vi "frequency_sweep_1.vi"() -> ()   [LabVIEW 2016]
uses:
  <instrlib>/niVNA/niVNA.llb/niVNA Fetch Sweep Measurement (DBL).vi
panel:
  in  "IF Bandwidth":dbl(ring)=1000.0 items=["10 Hz"=10.0, "30 Hz"=30.0, "100 Hz"=100.0, "300 Hz"=300.0, "1 KHz"=1000.0, "3 KHz"=3000.0, "10 KHz"=10000.0, "30 KHz"=30000.0]
  in  "Save Button":bool
  out "Status":string="Measurement Running..."
  out "Cursor":cluster{"x":dbl, "y":dbl} {"x" format="%.5f"; "y" format="%.5f"}
  out "Resource Name Out":refnum<k15>
  out "Error Out":errorcluster
  in  "Error In (no error)":errorcluster
  in  "Format":i32(ring) items=["Log Magnitude (dB)"=0, "Lin Magnitude"=1, "Phase (deg)"=2, "VSWR"=3, "Group Delay"=6]
  out "SpectrumGraph":cluster{"Numeric":dbl, "real":dbl}[](graph)
  in  "Value":i32(ring)=1 items=["Im", "Re", "Abs"]
  in  "S-parameter":i32(ring)=1 caption="Measurement" items=["S11", "S21"]
  in  "Exit Button":bool
  in  "Start Button":bool
  in  "Stop Button":bool
  in  "Output Power":dbl=1.0
  in  "Number of Points":i32=1024 min=1 max=3201
  in  "Stop Frequency":dbl=6000000000.0 min=10000000.0 max=6000000000.0 format="%#_6e"
  in  "Start Frequency":dbl=1000000000.0 min=10000000.0 max=6000000000.0 format="%#_6e"
  in  "Resource Name In":refnum<k15>="VNA_5630"
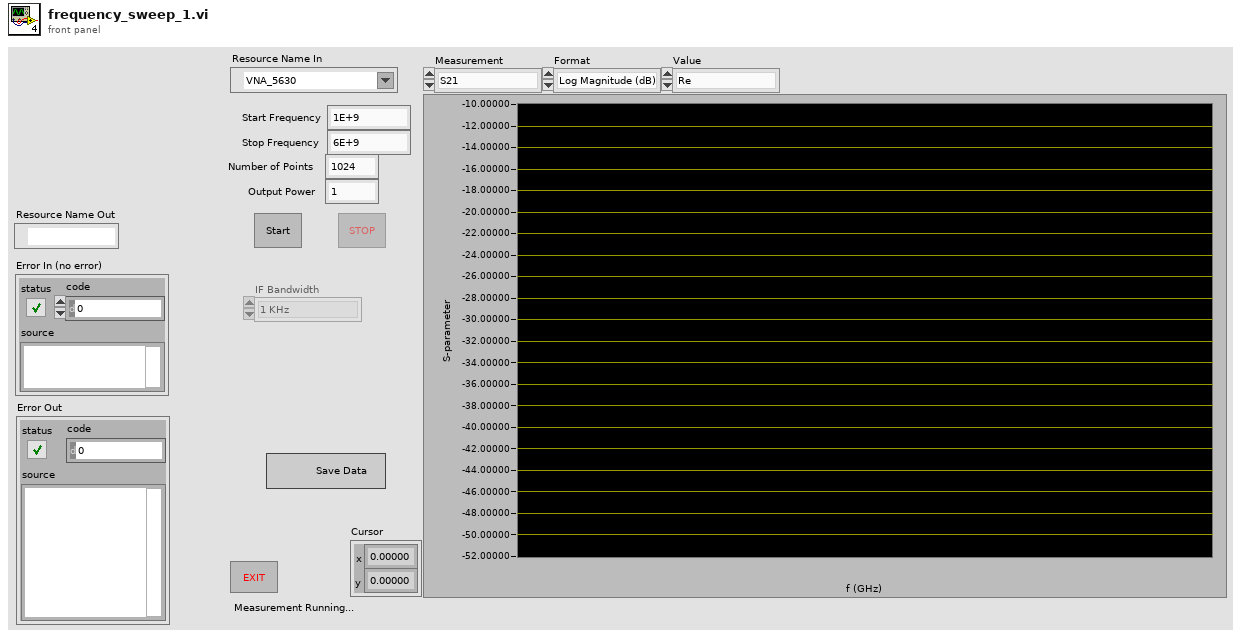
[diagram p1: front panel]
types:
  T1 = typedef "LVPoint32TypeDef.ctl" = cluster{"Horizontal":i32, "Vertical":i32}
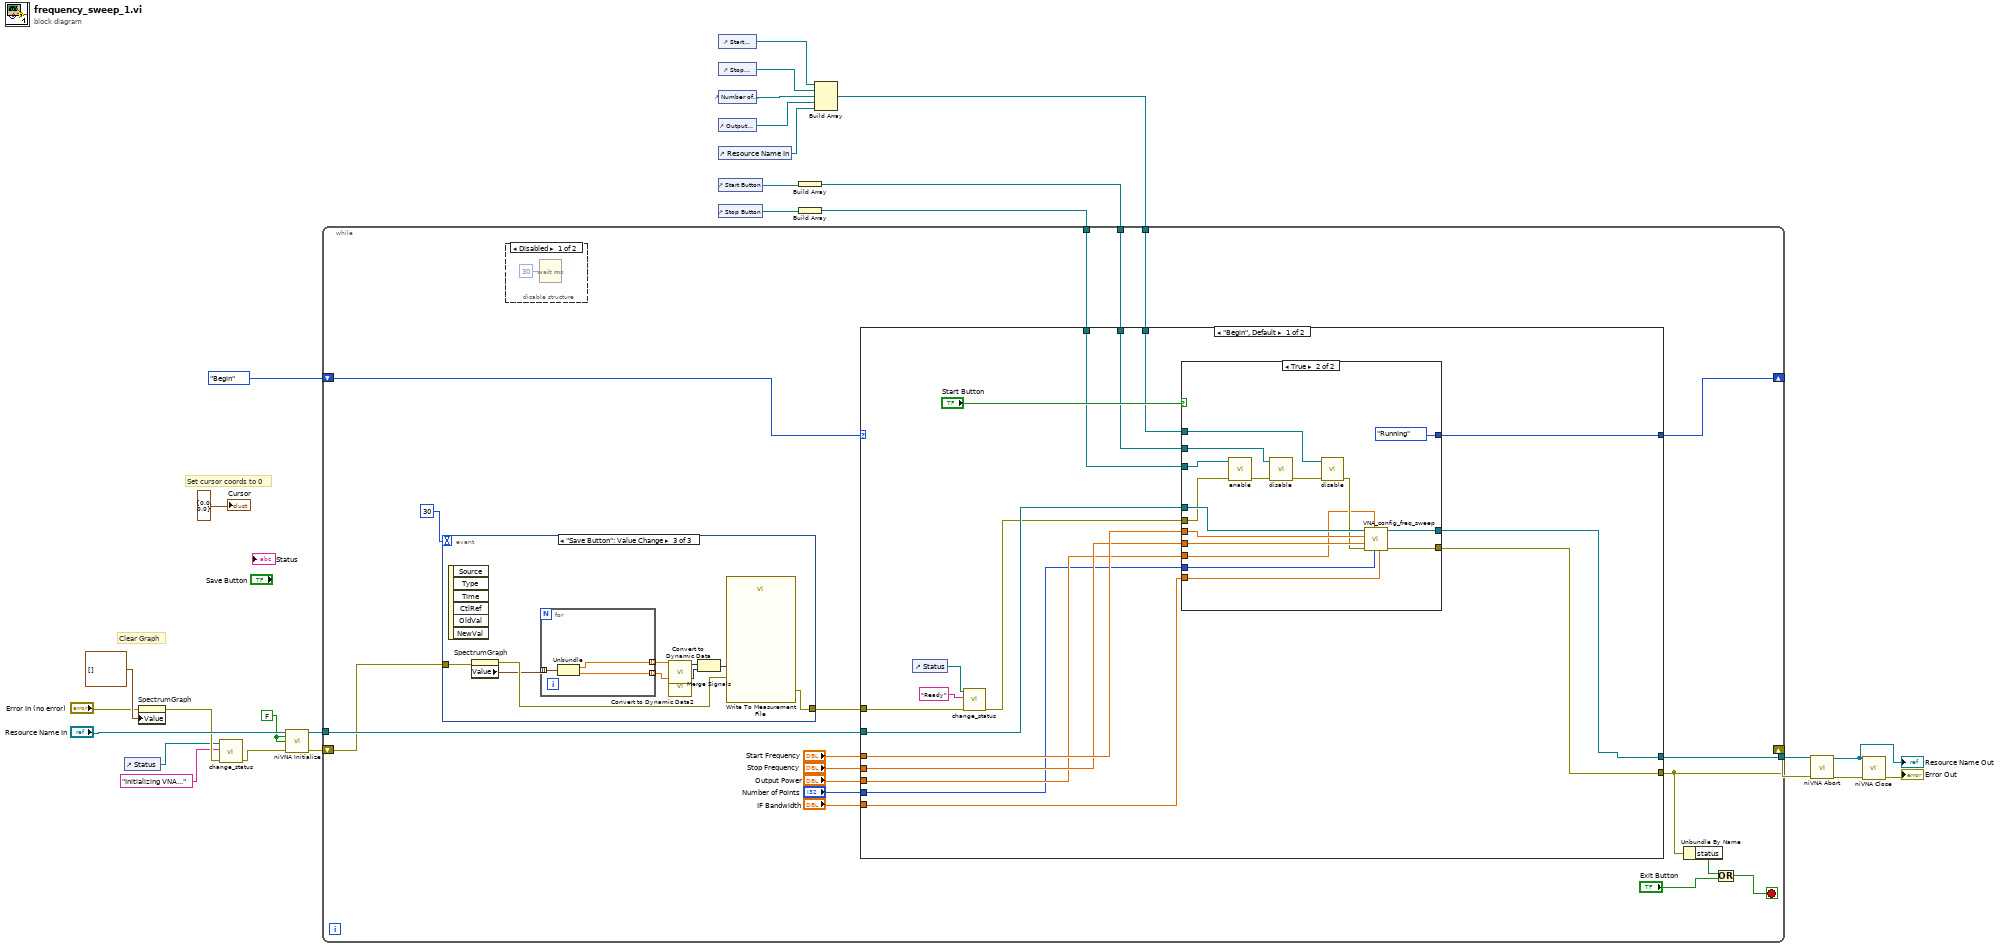
[diagram p0: block diagram]
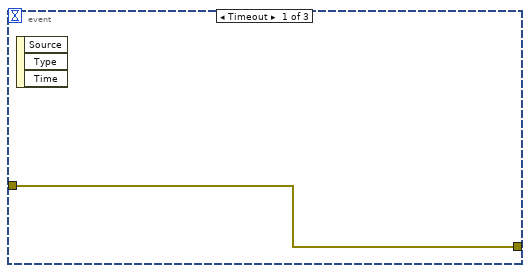
[diagram p3: hidden frame]
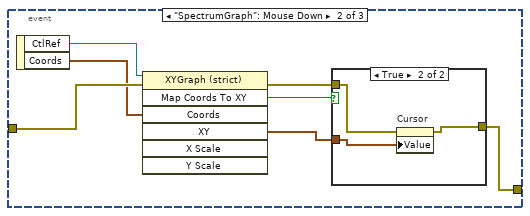
[diagram p4: hidden frame]
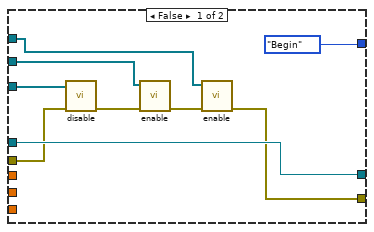
[diagram p6: hidden frame]
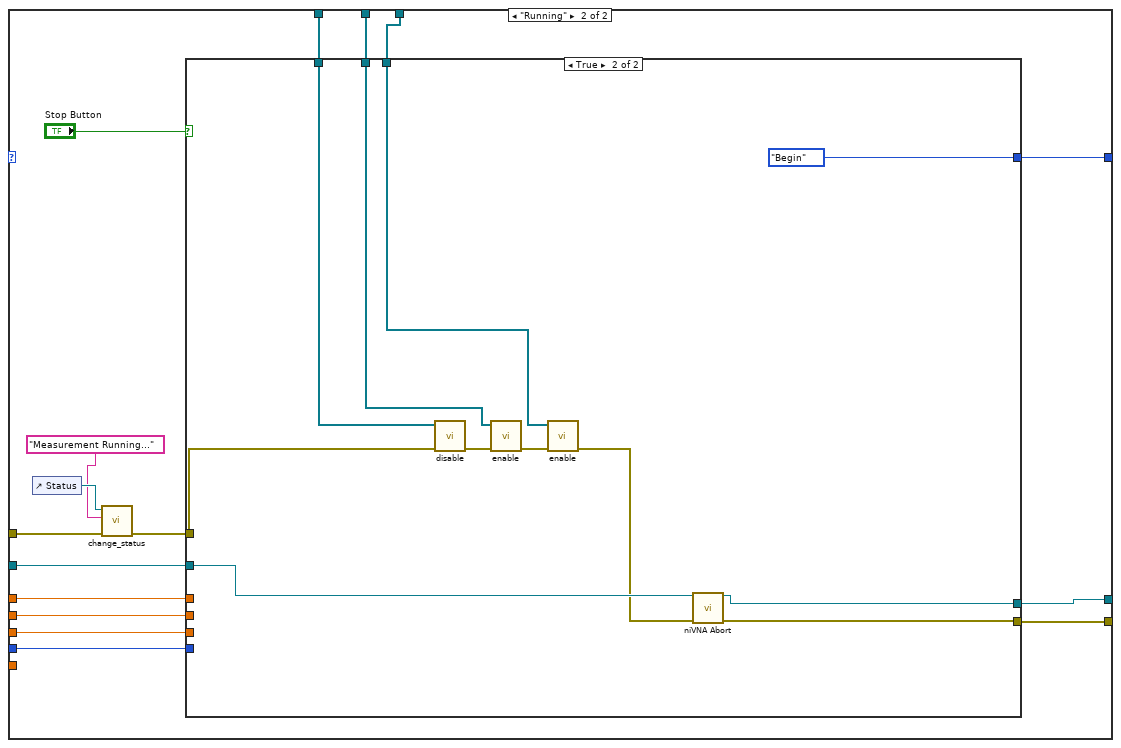
[diagram p7: hidden frame]
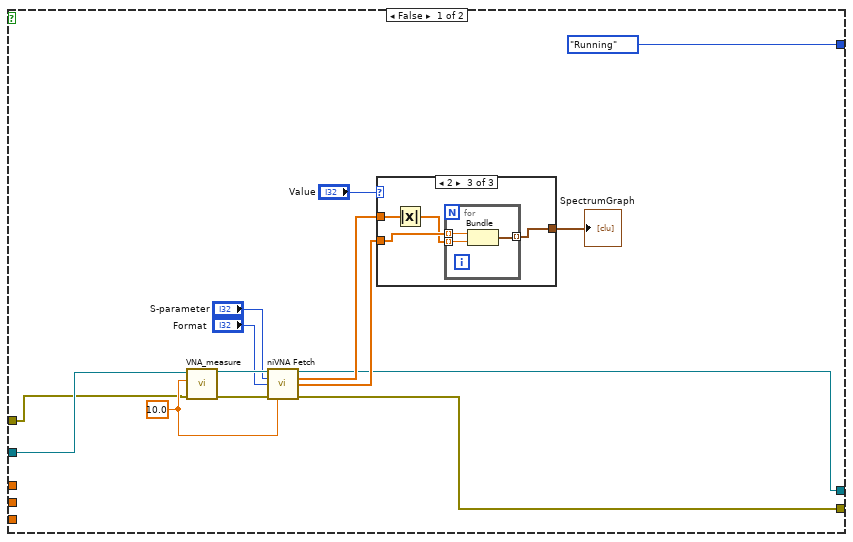
[diagram p8: hidden frame]
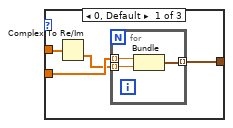
[diagram p9: hidden frame]
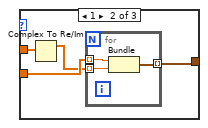
[diagram p10: hidden frame]
diagram:
  w7 = FALSE ("id query")
  # "Set cursor coords to 0"
  # "Clear Graph"
  n1 = control-ref of="Status"() -> (w1:refnum<vi>)
  n2 = property on="SpectrumGraph" class="XYGraph (strict)"(error in="Error In (no error)", "Value"=cluster{"Numeric":dbl, "real":dbl}[] [] ("SpectrumGraph")) -> (error out=w4:errorcluster)  [unwired: 1 in, 1 out]
  n3 = call "change_status.vi"("error in (no error)"=w4, "String"="Initializing VNA...", "String in"=w1) -> ("error out"=w3:errorcluster)  [unwired: 8 in]
  n4 = call <instrlib>:"niVNA Initialize.vi"("resource name"="Resource Name In", "id query"=w7, "reset"=w7, "error in"=w3) -> ("instrument handle"=w8:refnum<k15>, "error out"=w5:errorcluster)  [unwired: 10 in]
  n5 = control-ref of="Start Frequency"() -> (w27:refnum<vi>)
  n6 = control-ref of="Stop Frequency"() -> (w26:refnum<vi>)
  n7 = control-ref of="Number of Points"() -> (w25:refnum<vi>)
  n8 = control-ref of="Output Power"() -> (w24:refnum<vi>)
  n9 = control-ref of="Resource Name In"() -> (w23:refnum<vi>)
  n10 = control-ref of="Start Button"() -> (w19:refnum<vi>)
  n11 = control-ref of="Stop Button"() -> (w21:refnum<vi>)
  n12 = Build Array(w19) -> (w18:refnum<vi>[])
  n13 = Build Array(w21) -> (w20:refnum<vi>[])
  n14 = Build Array(w27, w26, w25, w24, w23) -> (w17:refnum<vi>[])
  n15 = while {
    shift-right: [w41] -> _
    shift-left: enum16{"Begin", "Running"}."Begin" -> [w46]
    tunnel: w20 -> [w37]
    tunnel: w18 -> [w35]
    tunnel: w17 -> [w34]
    tunnel: w8 -> [w33]
    tunnel: [w30] -> w6
    shift-right: [w36] -> w11
    shift-left: w5 -> [w29]
    stop <- w38 stop-if-true
    n16 = event shown="[2] \"Save Button\": Value Change" {
      selector: _ -> [_ _ _]
      dyn-events: _ -> [_ _ _]
      timeout: u32 30 ("milliseconds to wait") -> [_ _ _]
      tunnel: w29 -> [w48 w52 w67]
      tunnel: [w48 w51 w68] -> w32
      event Timeout {
        n17 = event-data() -> ()  [unwired: 1 in, 3 out]
      }
      event "SpectrumGraph": Mouse Down {
        n18 = event-data() -> ("CtlRef"=w49:refnum<vi>, "Coords"=w50:T1)  [unwired: 1 in]
        n19 = invoke on="Invoke Node" class="XYGraph (strict)" method="Map Coords To XY"(reference=w49, error in=w52, "Coords"=w50) -> (error out=w55:errorcluster, "Map Coords To XY"=w53:bool, "XY"=w54:cluster{"X":dbl, "Y":dbl})  [unwired: 4 in, 4 out]
        n20 = case shown="True" w53 {
          tunnel: w54 -> [_ w57]
          tunnel: w55 -> [w56 w59]
          tunnel: [w56 w58] -> w51
          frame False {
          }
          frame True {
            n21 = property on="Cursor" class="Clust (strict)"(error in=w59, "Value"=w57) -> (error out=w58:errorcluster)  [unwired: 1 in, 1 out]
          }
        }
      }
      event "Save Button": Value Change {
        n22 = event-data() -> ()  [unwired: 1 in, 6 out]
        n23 = property on="SpectrumGraph" class="XYGraph (strict)"(error in=w67) -> (error out=w66:errorcluster, "Value"=w65:cluster{"Numeric":dbl, "real":dbl}[])  [unwired: 1 in, 1 out]
        n24 = for {
          tunnel: w65 -> [w71] mode=indexing
          tunnel: [w70] -> w64 mode=indexing
          tunnel: [w69] -> w61 mode=indexing
          n25 = Unbundle(w71) -> ("Numeric"=w70:dbl, "real"=w69:dbl)
        }
        n26 = call "Convert to Dynamic Data"("Array"=w64) -> ("Dynamic Data Type"=w63:dynamicdata)  [unwired: 3 in]
        n27 = call "Convert to Dynamic Data2"("Array"=w61) -> ("Dynamic Data Type"=w60:dynamicdata)  [unwired: 3 in]
        n28 = Merge Signals(w63, w60) -> (w62:dynamicdata)
        n29 = call "Write To Measurement File"("Signals"=w62, "error in (no error)"=w66) -> ("error out"=w68:errorcluster)  [unwired: 15 in, 2 out]
      }
    }
    n30 = disable-structure shown="Disabled" {
      frame Disabled {
        n31 = Wait (ms)(milliseconds to wait=u32 30) -> ()  [unwired: 1 out]
      }
      frame Enabled {
      }
    }
    n32 = case shown="\"Begin\", Default" w46 {
      tunnel: w33 -> [w86 w127]
      tunnel: "Start Frequency" -> [w85 w126]
      tunnel: "Stop Frequency" -> [w84 w125]
      tunnel: "Output Power" -> [w83 w124]
      tunnel: "Number of Points" -> [w82 w123]
      tunnel: [w87 w128] -> w41
      tunnel: [w81 w121] -> w30
      tunnel: [w80 w122] -> w36
      tunnel: w37 -> [w79 w120]
      tunnel: w32 -> [w74 w115]
      tunnel: w35 -> [w78 w119]
      tunnel: w34 -> [w77 w118]
      tunnel: "IF Bandwidth" -> [w72 _]
      frame "Begin", Default {
        n33 = control-ref of="Status"() -> (w75:refnum<vi>)
        n34 = call "change_status.vi"("error in (no error)"=w74, "String"="Ready", "String in"=w75) -> ("error out"=w73:errorcluster)  [unwired: 8 in]
        n35 = case shown="True" "Start Button" {
          tunnel: [enum16{"Begin", "Running"}."Begin" enum16{"Begin", "Running"}."Running"] -> w87
          tunnel: w86 -> [w96 w112]
          tunnel: w85 -> [_ w111]
          tunnel: w84 -> [_ w110]
          tunnel: w83 -> [_ w99]
          tunnel: w82 -> [_ w109]
          tunnel: [w96 w108] -> w81
          tunnel: [w92 w107] -> w80
          tunnel: w79 -> [w95 w102]
          tunnel: w73 -> [w91 w101]
          tunnel: w78 -> [w90 w104]
          tunnel: w77 -> [w89 w103]
          tunnel: w72 -> [_ w98]
          frame False {
            n36 = call "disable.vi"("error in (no error)"=w91, "Array"=w95) -> ("error out"=w94:errorcluster)  [unwired: 9 in]
            n37 = call "enable.vi"("error in (no error)"=w94, "Array"=w90) -> ("error out"=w93:errorcluster)  [unwired: 9 in]
            n38 = call "enable.vi"("error in (no error)"=w93, "Array"=w89) -> ("error out"=w92:errorcluster)  [unwired: 9 in]
          }
          frame True {
            n39 = call "enable.vi"("error in (no error)"=w101, "Array"=w102) -> ("error out"=w100:errorcluster)  [unwired: 9 in]
            n40 = call "disable.vi"("error in (no error)"=w100, "Array"=w104) -> ("error out"=w106:errorcluster)  [unwired: 9 in]
            n41 = call "disable.vi"("error in (no error)"=w106, "Array"=w103) -> ("error out"=w105:errorcluster)  [unwired: 9 in]
            n42 = call "VNA_config_freq_sweep.vi"("IF Bandwidth"=w98, "Number of Points"=w109, "Output Power"=w99, "error in (no error)"=w105, "Stop Frequency"=w110, "Start Frequency"=w111, "Resource Name In"=w112) -> ("error out"=w107:errorcluster, "Resource Name Out"=w108:refnum<k15>)  [unwired: 3 in]
          }
        }
      }
      frame "Running" {
        n43 = control-ref of="Status"() -> (w117:refnum<vi>)
        n44 = call "change_status.vi"("error in (no error)"=w115, "String"="Measurement Running...", "String in"=w117) -> ("error out"=w114:errorcluster)  [unwired: 8 in]
        n45 = case shown="True" "Stop Button" {
          tunnel: [enum16{"Begin", "Running"}."Running" enum16{"Begin", "Running"}."Begin"] -> w128
          tunnel: w127 -> [w134 w174]
          tunnel: w126 -> [_ _]
          tunnel: w125 -> [_ _]
          tunnel: w124 -> [_ _]
          tunnel: w123 -> [_ _]
          tunnel: [w131 w165] -> w122
          tunnel: [w133 w173] -> w121
          tunnel: w114 -> [w130 w167]
          tunnel: w120 -> [_ w170]
          tunnel: w119 -> [_ w169]
          tunnel: w118 -> [_ w168]
          frame False {
            w139 = 10.0 ("timeout")
            n46 = call "VNA_measure.vi"("error in (no error)"=w130, "timeout"=w139, "Resource Name In"=w134) -> ("error out"=w140:errorcluster, "Resource Name Out"=w142:refnum<k15>)  [unwired: 7 in]
            n47 = call-poly <instrlib>:"niVNA Fetch.vi"("instrument handle"=w142, "measurement"="S-parameter", "format"="Format", "error in"=w140, "timeout"=w139) -> ("instrument handle out"=w133:refnum<k15>, "data"=w136:dbl[], "scale points"=w137:dbl[], "error out"=w131:errorcluster)  [unwired: 7 in]
            n48 = case shown="2" "Value" {
              tunnel: w137 -> [w145 w152 w159]
              tunnel: w136 -> [w147 w154 w161]
              tunnel: [w146 w153 w160] -> w132
              frame 0, Default {
                n49 = Complex To Re/Im(x + iy=w147) -> (y=w144:dbl[])  [unwired: 1 out]
                n50 = for {
                  tunnel: w145 -> [w150] mode=indexing
                  tunnel: [w149] -> w146 mode=indexing
                  tunnel: w144 -> [w148] mode=indexing
                  n51 = Bundle("Numeric"=w150, "Numeric"=w148) -> (w149:cluster{"Numeric":dbl, "Numeric":dbl})  [unwired: 1 in]
                }
              }
              frame 1 {
                n52 = Complex To Re/Im(x + iy=w154) -> (x=w151:dbl[])  [unwired: 1 out]
                n53 = for {
                  tunnel: [w157] -> w153 mode=indexing
                  tunnel: w151 -> [w156] mode=indexing
                  tunnel: w152 -> [w155] mode=indexing
                  n54 = Bundle("Numeric"=w155, "Numeric"=w156) -> (w157:cluster{"Numeric":dbl, "Numeric":dbl})  [unwired: 1 in]
                }
              }
              frame 2 {
                n55 = Absolute Value(x=w161) -> (abs(x)=w158:dbl[])
                n56 = for {
                  tunnel: w159 -> [w164] mode=indexing
                  tunnel: [w163] -> w160 mode=indexing
                  tunnel: w158 -> [w162] mode=indexing
                  n57 = Bundle("Numeric"=w164, "Numeric"=w162) -> (w163:cluster{"Numeric":dbl, "Numeric":dbl})  [unwired: 1 in]
                }
              }
            }
            "SpectrumGraph" <- w132
          }
          frame True {
            n58 = call "disable.vi"("error in (no error)"=w167, "Array"=w170) -> ("error out"=w172:errorcluster)  [unwired: 9 in]
            n59 = call "enable.vi"("error in (no error)"=w172, "Array"=w169) -> ("error out"=w171:errorcluster)  [unwired: 9 in]
            n60 = call "enable.vi"("error in (no error)"=w171, "Array"=w168) -> ("error out"=w166:errorcluster)  [unwired: 9 in]
            n61 = call <instrlib>:"niVNA Abort.vi"("instrument handle"=w174, "error in"=w166) -> ("instrument handle out"=w173:refnum<k15>, "error out"=w165:errorcluster)  [unwired: 12 in]
          }
        }
      }
    }
    n62 = Unbundle By Name(w36) -> ("status"=w40:bool)
    n63 = Or(x=w40, y="Exit Button") -> (x .or. y?=w38:bool)
  }
  n64 = call <instrlib>:"niVNA Abort.vi"("instrument handle"=w6, "error in"=w11) -> ("instrument handle out"=w10:refnum<k15>, "error out"=w12:errorcluster)  [unwired: 12 in]
  "Resource Name Out" <- w10
  n65 = call <instrlib>:"niVNA Close.vi"("instrument handle"=w10, "error in"=w12) -> ("error out"=→"Error Out":errorcluster)  [unwired: 13 in]
  "Cursor" <- cluster{"x":dbl, "y":dbl} {"x"=0.0, "y"=0.0} ("Cursor")
